vi "Process Session Exec.vi"(0 "command line":string, 1 "stop refnum":refnum<vi>, 2 "stdout refnum":refnum<vi>, 3 "stderr refnum":refnum<vi>, 5 "working directory":path, 7 "stdin":string, 9 "timeout (ms)":i32=-1, 11 "error in (no error)":errorcluster, 12 "merge output":bool) -> (4 "stdout":string, 6 "stderr":string, 8 "exit code":u32, 10 "timed out":bool, 15 "error out":errorcluster)   [LabVIEW 2013]
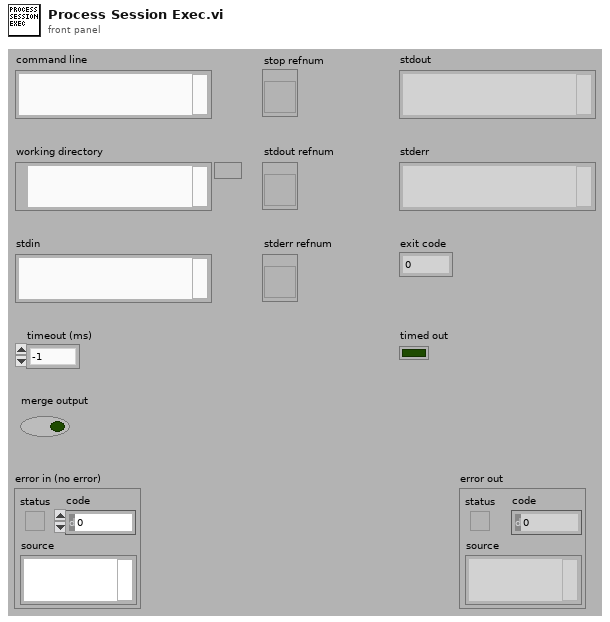
[diagram p1: front panel]
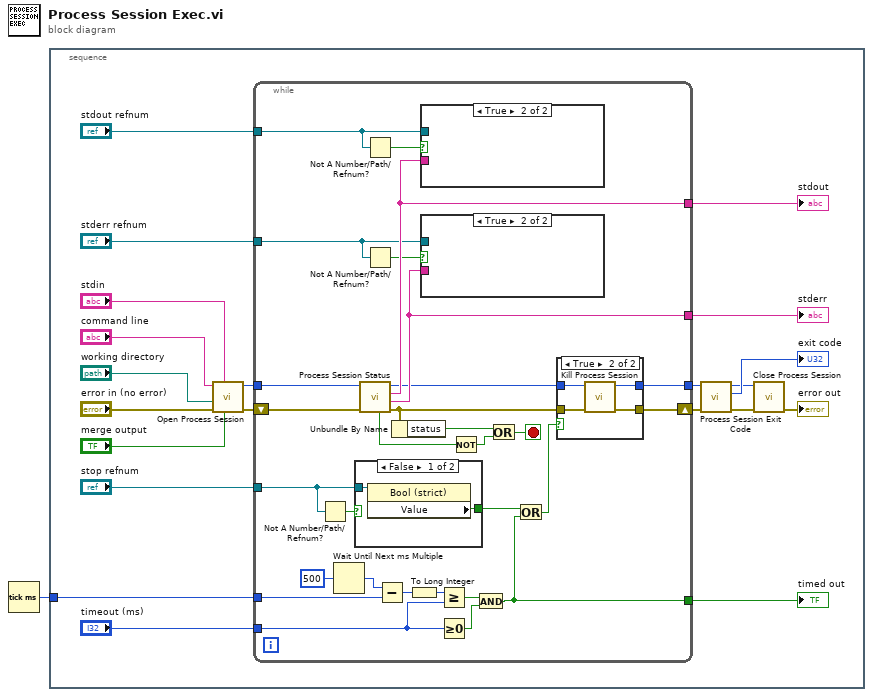
[diagram p0: block diagram]
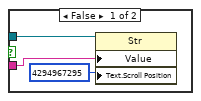
[diagram p3: hidden frame]
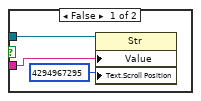
[diagram p4: hidden frame]
diagram:
  n1 = Tick Count (ms)() -> (millisecond timer value=w1:u32)
  n2 = stacked-sequence {
    tunnel: w1 -> [w11]
    frame #0 {
      n3 = call "Open Process Session.vi"("merge output"="merge output", "stdin"="stdin", "error in (no error)"="error in (no error)", "working directory"="working directory", "command line"="command line") -> ("error out"=w22:errorcluster, "session ID"=w20:i32)  [unwired: 5 in]
      n4 = while {
        tunnel: w20 -> [w35]
        shift-right: [w31] -> w14
        shift-left: w22 -> [w34]
        tunnel: [w30] -> w15
        tunnel: "stop refnum" -> [w50]
        tunnel: "stdout refnum" -> [w44]
        tunnel: "stderr refnum" -> [w29]
        tunnel: w11 -> [w43]
        tunnel: "timeout (ms)" -> [w40]
        tunnel: [w37] -> w6
        tunnel: [w36] -> w5
        tunnel: [w26] -> w3
        stop <- w49 stop-if-true
        n5 = Not A Number/Path/Refnum?(number/path/refnum=w50) -> (NaN/Path/Refnum?=w51:bool)
        n6 = Wait Until Next ms Multiple(millisecond multiple=u32 500) -> (millisecond timer value=w24:u32)
        n7 = case shown="False" w51 {
          tunnel: w50 -> [w65 _]
          tunnel: [w64 _] -> w25
          frame False {
            n8 = property class="Bool (strict)"(reference=w65) -> ("Value"=w64:bool)  [unwired: 1 in, 2 out]
          }
          frame True {
          }
        }
        n9 = call "Process Session Status.vi"("error in (no error)"=w34, "session ID in"=w35) -> ("error out"=w32:errorcluster, "stderr"=w36:string, "stdout"=w37:string, "session ID out"=w33:i32, "running"=w47:bool)  [unwired: 5 in]
        n10 = Not A Number/Path/Refnum?(number/path/refnum=w44) -> (NaN/Path/Refnum?=w45:bool)
        n11 = Not A Number/Path/Refnum?(number/path/refnum=w29) -> (NaN/Path/Refnum?=w28:bool)
        n12 = Subtract(x=w24, y=w43) -> (x-y=w42:u32)
        n13 = Unbundle By Name(w32) -> ("status"=w48:bool)
        n14 = To Long Integer(number=w42) -> (32bit integer=w41:i32)
        n15 = case shown="True" w45 {
          tunnel: w37 -> [w62 _]
          tunnel: w44 -> [w63 _]
          frame False {
            n16 = property class="Str"(reference=w63, "Value"=w62, "Text.Scroll Position"=u32 4294967295) -> ()  [unwired: 1 in, 2 out]
          }
          frame True {
          }
        }
        n17 = case shown="True" w28 {
          tunnel: w36 -> [w59 _]
          tunnel: w29 -> [w60 _]
          frame False {
            n18 = property class="Str"(reference=w60, "Value"=w59, "Text.Scroll Position"=u32 4294967295) -> ()  [unwired: 1 in, 2 out]
          }
          frame True {
          }
        }
        n19 = Greater Or Equal?(x=w41, y=w40) -> (x >= y?=w39:bool)
        n20 = Greater Or Equal To 0?(x=w40) -> (x >= 0?=w38:bool)
        n21 = Not(x=w47) -> (.not. x?=w46:bool)
        n22 = And(x=w39, y=w38) -> (x .and. y?=w26:bool)
        n23 = Or(x=w48, y=w46) -> (x .or. y?=w49:bool)
        n24 = Or(x=w25, y=w26) -> (x .or. y?=w27:bool)
        n25 = case shown="True" w27 {
          tunnel: w32 -> [w52 w55]
          tunnel: w33 -> [w53 w57]
          tunnel: [w53 w56] -> w30
          tunnel: [w52 w54] -> w31
          frame False {
          }
          frame True {
            n26 = call "Kill Process Session .vi"("error in (no error)"=w55, "session ID in"=w57) -> ("error out"=w54:errorcluster, "session ID out"=w56:i32)  [unwired: 8 in]
          }
        }
      }
      "stdout" <- w6
      "stderr" <- w5
      "timed out" <- w3
      n27 = call "Process Session Exit Code.vi"("error in (no error)"=w14, "session ID in"=w15) -> ("error out"=w13:errorcluster, "exit code"=→"exit code":u32, "session ID out"=w4:i32)  [unwired: 7 in]
      n28 = call "Close Process Session.vi"("error in (no error)"=w13, "session ID"=w4) -> ("error out"=→"error out":errorcluster)  [unwired: 9 in]
    }
  }
